vi "Read Attributes.vi"(11 "UpdateTimeToParent Msg":refnum<class "UpdateTimeToParent Msg.lvclass">) -> (2 "Payload":cluster{"ElapsedTime":i32})   [LabVIEW 2020, in "Timer_Event.lvlib" / "UpdateTimeToParent Msg.lvclass"]
uses:
  UpdateTimeToParent Msg.lvclass
  UpdateTimeToParent Msg.lvclass/UpdateTimeToParent Msg.ctl
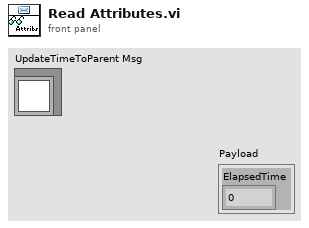
[diagram p1: front panel]
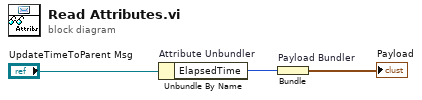
[diagram p0: block diagram]
diagram:
  n1 = Unbundle By Name "Attribute Unbundler"("UpdateTimeToParent Msg") -> ("ElapsedTime"=w1:i32)
  n2 = Bundle "Payload Bundler"("ElapsedTime"=w1) -> (→"Payload":cluster{"ElapsedTime":i32})  [unwired: 1 in]
